vi "Open FPGA Reference.vi"(8 "Error In":errorcluster, 11 "Settings.Compiled":T18={"Name"="", "RIO.Address"="", "Bitfile.Path"=path "", "Injectors.Count"=0, "Injectors.Settings"=[], "Waveform.Refs"=[], "VS.Registers"={"Block Data refs"=[], "Values"=[]}, "Registers"=[], "Timing.Registers"=[], "Mux.Register"={"Name"="", "Data Type"=enum."<Null>", "Default Value"=variant(dbl 0.0)}, "Groups.Settings"=[]} {"Mux.Register"."Data Type" format="%.0x"; "Registers"."Register"."Data Type" format="%.0x"; "VS.Registers"."Block Data refs"."Data Reference" format="%.0x"}) -> (0 "Error Out":errorcluster, 2 "Async Parameters":T1, 3 "Inline State Data out":T13 {"VS.Registers"."Data Reference" format="%.0x"; "FPGA.Registers"."Data Type" format="%.0x"})   [LabVIEW 2019, in "Fuel Injector Analysis Addon Engine.lvlib"]
uses:
  Fuel Injector Analysis Addon Engine.lvlib
  <vilib>/rvi/interface/nirviMethod/nirviMethod.xnode
  <vilib>/rvi/errors/niLvFpgaMergeErrorWithErrorCode.vi
  <vilib>/NI/LVFPGA Adv Session Resources/OpenByName.xnode
  Addon Shared/SubVIs/Constants.vi
  Addon Shared/Fuel Injector Analysis Addon Shared.lvlib
  <vilib>/NI/NIVS Inline Async API/_Data Access Engine/Access Type Classes/Write/Write.lvclass
  <vilib>/NI/NIVS Inline Async API/_Data Access Engine/Access Type Classes/Read/Read.lvclass
  <vilib>/NI VeriStand/Custom Device Waveform API/Single Waveform Write (DBL)/Single Waveform Write (DBL).lvclass
  <vilib>/NI VeriStand/Custom Device API/Waveform Data Reference.ctl
  <vilib>/NI VeriStand/Custom Device API/Custom Device API.lvlib
  Addon Shared/Types/Injector info.ctl
  Types/Async Parameters.ctl
  <vilib>/NI/NIVS Inline Async API/_VS Inline Async API/VS Inline Async API/VS Inline Async API.lvclass
  Addon Shared/Types/FPGA Data Types.ctl
  Types/FPGA Refs.ctl
  <vilib>/NI VeriStand/Custom Device API/Data Reference.ctl
  <vilib>/NI VeriStand/Custom Device API/Block Data Reference.ctl
  Types/Inline State Data.ctl
  <vilib>/FPGAPlugInAG/Dynamic/niLvFpga_ConfigureFifo_Dynamic.vi
  <vilib>/FPGAPlugInAG/Dynamic/niLvFpga_StartFifo_Dynamic.vi
  Addon Shared/Types/Analysis.Channels.Select.ctl
  <vilib>/NI/NIVS Inline Async API/_Data Access Engine/Data Access Engine/Types/Write.DVR.ctl
  <vilib>/NI/NIVS Inline Async API/_Data Access Engine/Data Access Engine/Data Access Engine.lvclass
  <vilib>/NI/NIVS Inline Async API/_Data Access Engine/Data Access Engine/Types/Read.DVR.ctl
  Addon Shared/Types/Stage.Transition.Types.ctl
  Addon Shared/Types/Stage.PullIn.Types.ctl
  Addon Shared/Types/Stage.Parameters.ctl
  Addon Shared/Types/Shot.Parameters.ctl
  Types/Injector.State.ctl
  Addon Shared/Types/Compiled.Group.WaveformRefs.ctl
  <vilib>/NI/LVFPGA Adv Session Resources/OpenByNameSubVI.vi
  <vilib>/NI/LVFPGA Adv Session Resources/LVFPGAAdvSessionResources.lvlib
  Addon Shared/Types/Register.Info.ctl
  Addon Shared/Types/VS.Register.Info.ctl
  Addon Shared/Types/Compiled.Settings.ctl
  Addon Shared/Types/Compiled.Group.Timing.ctl
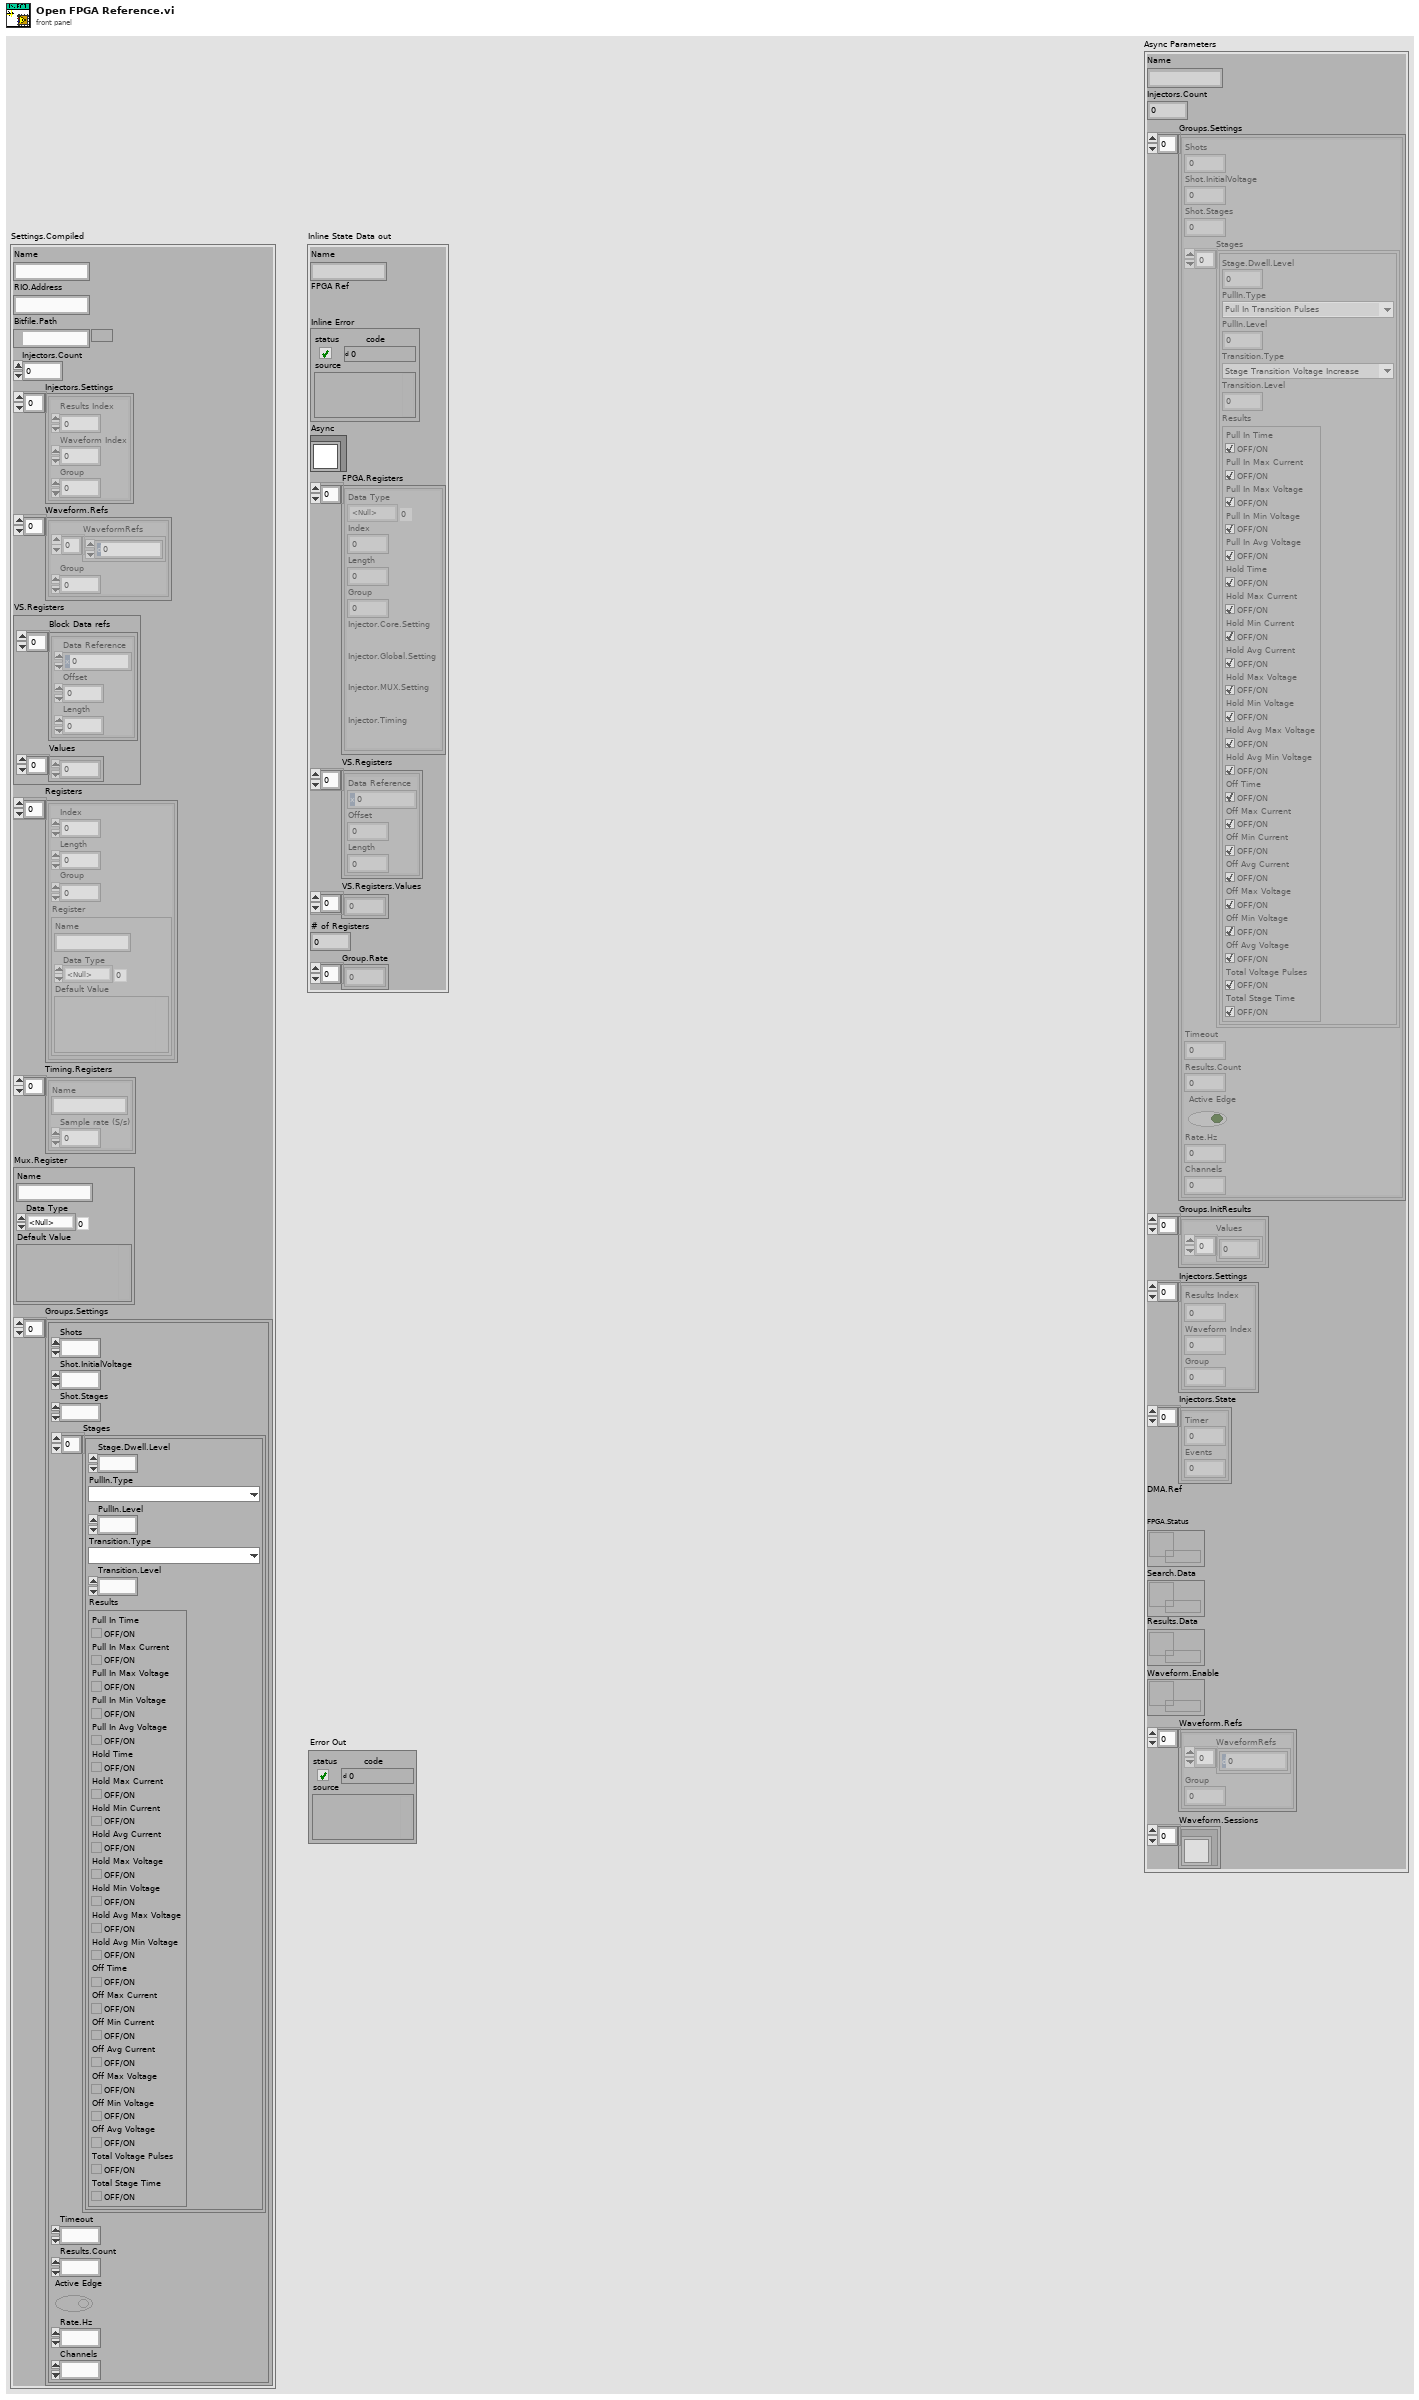
[diagram p1: front panel]
types:
  T1 = typedef "Fuel Injector Analysis Addon Engine.lvlib/Async Parameters.ctl" = cluster{"Name":string, "Injectors.Count":u8, "Groups.Settings":T2[], "Groups.InitResults":cluster{"Values":dbl[]}[], "Injectors.Settings":T7[], "Injectors.State":T8[], "DMA.Ref":refnum<k20>, "FPGA.Status":T9, "Search.Data":T10, "Results.Data":T9, "Waveform.Enable":T10, "Waveform.Refs":T11[], "Waveform.Sessions":refnum<class "Single Waveform Write (DBL).lvclass">[]}
  T2 = typedef "Fuel Injector Analysis Addon Shared.lvlib/Shot.Parameters.ctl" = cluster{"Shots":u32, "Shot.InitialVoltage":dbl, "Shot.Stages":u32, "Stages":T3[], "Timeout":dbl, "Results.Count":i32, "Active Edge":bool, "Rate.Hz":u32, "Channels":u32}
  T3 = typedef "Fuel Injector Analysis Addon Shared.lvlib/Stage.Parameters.ctl" = cluster{"Stage.Dwell.Level":dbl, "PullIn.Type":T4, "PullIn.Level":dbl, "Transition.Type":T5, "Transition.Level":dbl, "Results":T6}
  T4 = typedef "Fuel Injector Analysis Addon Shared.lvlib/Stage.PullIn.Types.ctl" = enum8{"Pull In Transition Pulses", "Pull In Transition Current Drop"}
  T5 = typedef "Fuel Injector Analysis Addon Shared.lvlib/Stage.Transition.Types.ctl" = enum8{"Stage Transition Inactive Time", "Stage Transition Voltage Increase", "Stage Transition Current Decrease", "Stage Transition Active Time"}
  T6 = typedef "Fuel Injector Analysis Addon Shared.lvlib/Analysis.Channels.Select.ctl" = cluster{"Pull In Time":bool, "Pull In Max Current":bool, "Pull In Max Voltage":bool, "Pull In Min Voltage":bool, "Pull In Avg Voltage":bool, "Hold Time":bool, "Hold Max Current":bool, "Hold Min Current":bool, "Hold Avg Current":bool, "Hold Max Voltage":bool, "Hold Min Voltage":bool, "Hold Avg Max Voltage":bool, "Hold Avg Min Voltage":bool, "Off Time":bool, "Off Max Current":bool, "Off Min Current":bool, "Off Avg Current":bool, "Off Max Voltage":bool, "Off Min Voltage":bool, "Off Avg Voltage":bool, "Total Voltage Pulses":bool, "Total Stage Time":bool}
  T7 = typedef "Fuel Injector Analysis Addon Shared.lvlib/Injector info.ctl" = cluster{"Results Index":i32, "Waveform Index":i32, "Group":u16}
  T8 = typedef "Fuel Injector Analysis Addon Engine.lvlib/Injector.State.ctl" = cluster{"Timer":u32, "Events":u64}
  T9 = typedef "Data Access Engine.lvlib/Data Access Engine.lvclass/Write.DVR.ctl" = refnum<data-value>
  T10 = typedef "Data Access Engine.lvlib/Data Access Engine.lvclass/Read.DVR.ctl" = refnum<data-value>
  T11 = typedef "Fuel Injector Analysis Addon Shared.lvlib/Compiled.Group.WaveformRefs.ctl" = cluster{"WaveformRefs":T12[], "Group":i32}
  T12 = typedef "Custom Device API.lvlib/Waveform Data Reference.ctl" = i32
  T13 = typedef "Fuel Injector Analysis Addon Engine.lvlib/Inline State Data.ctl" = cluster{"Name":string, "FPGA Ref":refnum<k20>, "Inline Error":errorcluster, "Async":refnum<class "VS Inline Async API.lvclass">, "FPGA.Registers":T14[], "VS.Registers":T16[], "VS.Registers.Values":dbl[], "# of Registers":u32, "Group.Rate":u32[]}
  T14 = typedef "Fuel Injector Analysis Addon Engine.lvlib/FPGA Refs.ctl" = cluster{"Data Type":T15, "Index":i32, "Length":i32, "Group":i32, "Injector.Core.Setting":refnum<k20>, "Injector.Global.Setting":refnum<k20>, "Injector.MUX.Setting":refnum<k20>, "Injector.Timing":refnum<k20>}
  T15 = typedef "Fuel Injector Analysis Addon Shared.lvlib/FPGA Data Types.ctl" = enum8{"<Null>", "Injector.Core.Setting", "Injector.Global.Setting", "Injector.Mux.Setting", "Injector.Timing"}
  T16 = typedef "Custom Device API.lvlib/Block Data Reference.ctl" = cluster{"Data Reference":T17, "Offset":u64, "Length":u64}
  T17 = typedef "Custom Device API.lvlib/Data Reference.ctl" = i32
  T18 = typedef "Fuel Injector Analysis Addon Shared.lvlib/Compiled.Settings.ctl" = cluster{"Name":string, "RIO.Address":string, "Bitfile.Path":path, "Injectors.Count":u32, "Injectors.Settings":T7[], "Waveform.Refs":T11[], "VS.Registers":cluster{"Block Data refs":T16[], "Values":dbl[]}, "Registers":T19[], "Timing.Registers":T21[], "Mux.Register":T20, "Groups.Settings":T2[]}
  T19 = typedef "Fuel Injector Analysis Addon Shared.lvlib/VS.Register.Info.ctl" = cluster{"Index":i32, "Length":i32, "Group":i32, "Register":T20}
  T20 = typedef "Fuel Injector Analysis Addon Shared.lvlib/Register.Info.ctl" = cluster{"Name":string, "Data Type":T15, "Default Value":variant}
  T21 = typedef "Fuel Injector Analysis Addon Shared.lvlib/Compiled.Group.Timing.ctl" = cluster{"Name":string, "Sample rate (S/s)":u32}
  T22 = cluster{"Name":string, "Depth":u32, "Write? (Deprecated:Use Implementation)":bool, "Physical Channel":u32, "Base Address":u32, "Data Width":u32, "Data Type":enum32{"Boolean", "I8", "I16", "I32", "I64", "U8", "U16", "U32", "U64", "FXP", "CustomControl", "SGL"}, "FXP Properties":variant, "Write Window Address":u32, "Implementation":enum16{"niFpgaTargetToHost", "niFpgaHostToTarget", "niFpgaPeerToPeerWriter", "niFpgaPeerToPeerReader", "niCoreTargetToHost", "niCoreHostToTarget"}, "Control Set":u32}[]
  T23 = cluster{"Name":string, "type":variant, "indicator?":bool}[]
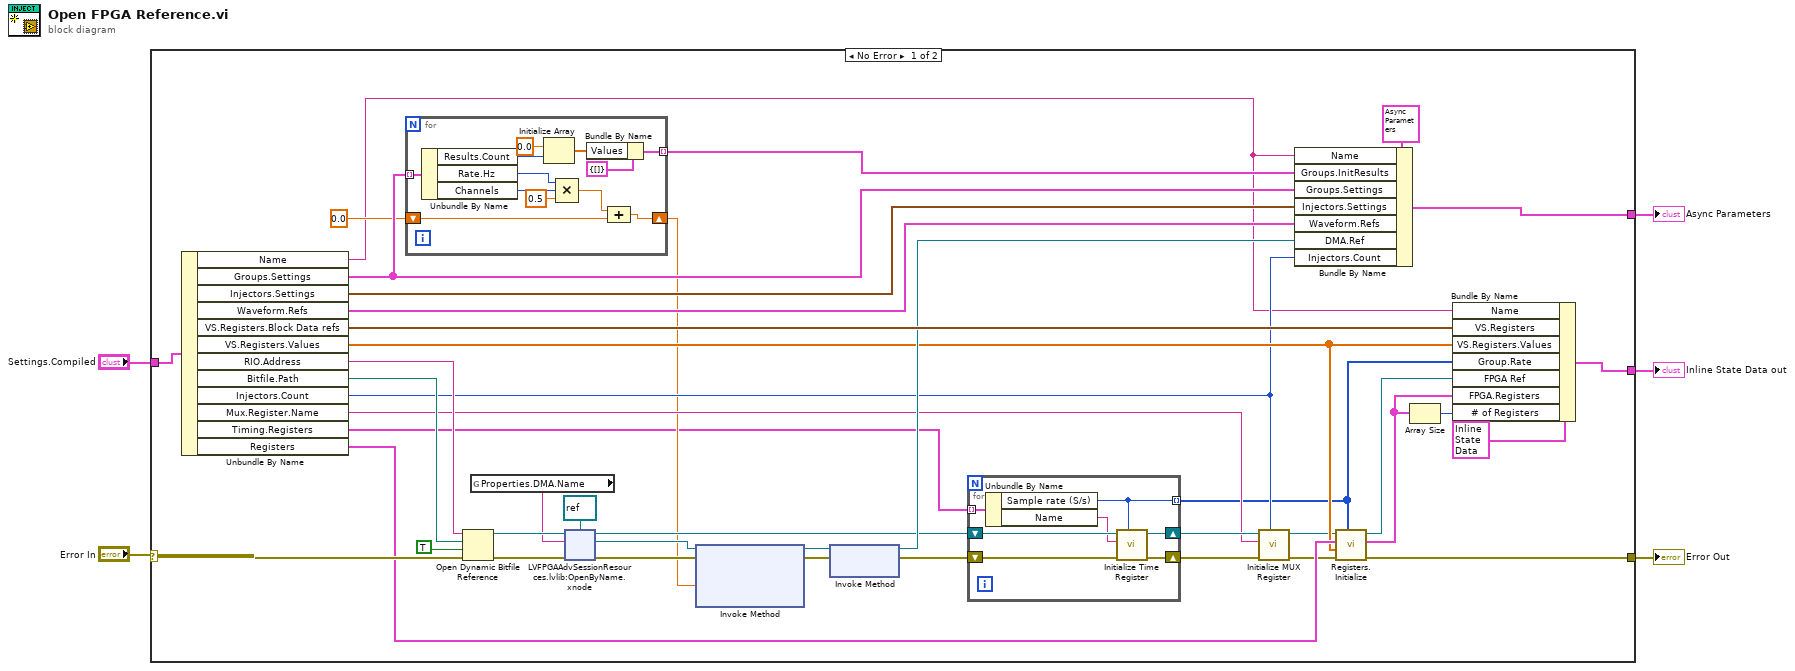
[diagram p0: block diagram]
diagram:
  n1 = case shown="No Error" "Error In" {
    selector: "Error In" -> [w46 w80]
    tunnel: [w35 w80] -> w4
    tunnel: "Settings.Compiled" -> [w30 _]
    tunnel: [w31 _] -> w2
    tunnel: [w24 _] -> w1
    frame No Error {
      n2 = Unbundle By Name(w30) -> ("Name"=w6:string, "Groups.Settings"=w13:T2[], "Injectors.Settings"=w26:T7[], "Waveform.Refs"=w27:T11[], "VS.Registers.Block Data refs"=w29:T16[], "VS.Registers.Values"=w19:dbl[], "RIO.Address"=w44:string, "Bitfile.Path"=w45:path, "Injectors.Count"=w11:u32, "Mux.Register.Name"=w14:string, "Timing.Registers"=w8:T21[], "Registers"=w34:T19[])
      n3 = for {
        tunnel: [w61] -> w12 mode=indexing
        tunnel: w13 -> [w65] mode=indexing
        shift-right: [w56] -> w9
        shift-left: 0.0 -> [w55]
        n4 = Unbundle By Name(w65) -> ("Results.Count"=w64:i32, "Rate.Hz"=w59:u32, "Channels"=w58:u32)
        n5 = Initialize Array(0.0, w64) -> (w62:dbl[])
        n6 = Compound Arithmetic op=MULTIPLY(w59, w58, 0.5 ("value")) -> (w57:dbl)
        n7 = Bundle By Name(cluster=cluster{"Values":dbl[]} {"Values"=[]} ("Values"), "Values"=w62) -> (w61:cluster{"Values":dbl[]})
        n8 = Compound Arithmetic op=ADD(w57, w55) -> (w56:dbl)
      }
      n9 = Open Dynamic Bitfile Reference(0:w44, 1:w45, 2:TRUE ("Run When Loaded"), 3:w46) -> (5:w37:refnum<k20>, 8:w38:errorcluster)  [unwired: 1 in]
      n10 = global read "Constants.vi" "Properties.DMA.Name"() -> (w36:string)
      n11 = xnode "LVFPGAAdvSessionResources.lvlib:OpenByName.xnode"("FPGA VI Reference in"=w37, "Resource name in"=w36, "Single resource reference type in"=refnum<k20> refnum, "Error in"=w38) -> ("Single resource reference out"=w39:refnum<k20>, "Error out"=w40:errorcluster, "FPGA VI Reference out"=w20:refnum<k20>)
      n12 = xnode "Invoke Method"("FPGA VI Reference In"=w39, "error in"=w40, "Requested Depth"=w9) -> ("FPGA VI Reference Out"=w42:refnum<k20>, "error out"=w41:errorcluster)  [unwired: 1 out]
      n13 = xnode "Invoke Method"("FPGA VI Reference In"=w42, "error in"=w41) -> ("FPGA VI Reference Out"=w28:refnum<k20>, "error out"=w21:errorcluster)
      n14 = for {
        shift-right: [w52] -> w18
        shift-left: w21 -> [w54]
        shift-right: [w51] -> w15
        shift-left: w20 -> [w53]
        tunnel: w8 -> [w50] mode=indexing
        tunnel: [w48] -> w7 mode=indexing
        n15 = Unbundle By Name(w50) -> ("Sample rate (S/s)"=w48:u32, "Name"=w49:string)
        n16 = call "Initialize Time Register.vi"("Sample rate (Hz)"=w48, "error in (no error)"=w54, "Name"=w49, "FPGA Ref"=w53) -> ("error out"=w52:errorcluster, "FPGA Ref out"=w51:refnum<k20>)  [unwired: 6 in]
      }
      n17 = call "Initialize MUX Register.vi"("# of Injectors"=w11, "error in (no error)"=w18, "Name"=w14, "FPGA Ref"=w15) -> ("error out"=w17:errorcluster, "FPGA Ref out"=w16:refnum<k20>)  [unwired: 6 in]
      n18 = Bundle By Name(cluster=T1 {"Name"="", "Injectors.Count"=0, "Groups.Settings"=[], "Groups.InitResults"=[], "Injectors.Settings"=[], "Injectors.State"=[], "DMA.Ref"=refnum, "FPGA.Status"=refnum, "Search.Data"=refnum, "Results.Data"=refnum, "Waveform.Enable"=refnum, "Waveform.Refs"=[], "Waveform.Sessions"=[]} ("Async Parameters"), "Name"=w6, "Groups.InitResults"=w12, "Groups.Settings"=w13, "Injectors.Settings"=w26, "Waveform.Refs"=w27, "DMA.Ref"=w28, "Injectors.Count"=w11) -> (w24:T1)
      n19 = call "Registers.Initialize.vi"("Group.Rate"=w7, "error in (no error)"=w17, "Values"=w19, "Registers"=w34, "FPGA Ref"=w16) -> ("error out"=w35:errorcluster, "Registers Ref"=w23:T14[], "FPGA Ref out"=w25:refnum<k20>)  [unwired: 4 in]
      n20 = Array Size(array=w23) -> (size(s)=w22:i32)
      n21 = Bundle By Name(cluster=T13 {"Name"="", "FPGA Ref"=refnum, "Inline Error"={"status"=FALSE, "code"=0, "source"=""}, "Async"=refnum, "FPGA.Registers"=[], "VS.Registers"=[], "VS.Registers.Values"=[], "# of Registers"=0, "Group.Rate"=[]} ("Inline State Data out"), "Name"=w6, "VS.Registers"=w29, "VS.Registers.Values"=w19, "Group.Rate"=w7, "FPGA Ref"=w25, "FPGA.Registers"=w23, "# of Registers"=w22) -> (w31:T13)
    }
    frame Error {
    }
  }
  "Error Out" <- w4
  "Inline State Data out" <- w2
  "Async Parameters" <- w1
